vi "TDT-Wait For Buffer Space.vi"(0 "RPcox":refnum<k7>, 5 "Next Buffer":i32, 7 "Tag":string="ch2Index", 9 "Buffer Length":i32, 11 "error in (no error)":errorcluster, 12 "Timeout (ms)":i32=5000) -> (4 "RPcox Out":refnum<k7>, 6 "Next Buffer thru":i32, 15 "error out":errorcluster)   [LabVIEW 2020]
uses:
  TDT-Globals.vi
panel:
  out "Available":bool
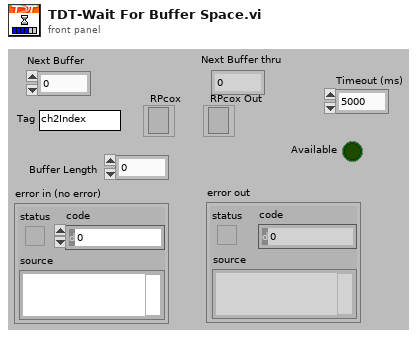
[diagram p1: front panel]
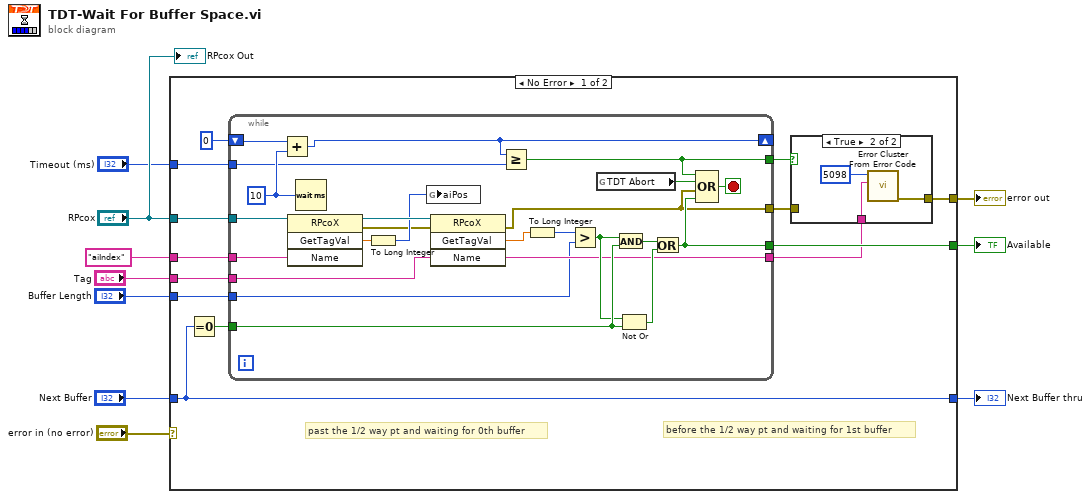
[diagram p0: block diagram]
diagram:
  n1 = case shown="No Error" "error in (no error)" {
    selector: "error in (no error)" -> [_ w52]
    tunnel: [w13 w52] -> w9
    tunnel: "RPcox" -> [w23 _]
    tunnel: "Buffer Length" -> [w22 _]
    tunnel: "Next Buffer" -> [w19 _]
    tunnel: [w20 _] -> w6
    tunnel: [w19 _] -> w5
    tunnel: "Tag" -> [w18 _]
    tunnel: "Timeout (ms)" -> [w16 _]
    tunnel: "aiIndex" ("format string") -> [w12 _]
    frame No Error {
      # "before the 1/2 way pt and waiting for 1st buffer"
      # "past the 1/2 way pt and waiting for 0th buffer"
      n2 = Equal To 0?(x=w19) -> (x = 0?=w21:bool)
      n3 = while {
        tunnel: w23 -> [w33]
        tunnel: w22 -> [w36]
        tunnel: w21 -> [w49]
        tunnel: [w45] -> w20
        tunnel: w18 -> [w43]
        shift-right: [w40] -> _
        shift-left: 0 -> [w42]
        tunnel: w16 -> [w39]
        tunnel: [w38] -> w15
        tunnel: [w37] -> w14
        tunnel: w12 -> [w32]
        tunnel: [w28] -> w11
        stop <- w44 stop-if-true
        w41 = u32 10 ("milliseconds to wait")
        n4 = Add(x=w42, y=w41) -> (x+y=w40:u32)
        n5 = invoke class="RPcoX" method="GetTagVal"(reference=w33, "Name"=w32) -> (reference out=w34:refnum<k7>, error out=w29:errorcluster, "GetTagVal"=w30:sgl)  [unwired: 2 in, 1 out]
        n6 = Wait (ms)(milliseconds to wait=w41) -> ()  [unwired: 1 out]
        n7 = To Long Integer(number=w30) -> (32bit integer=w31:i32)
        n8 = global write "TDT-Globals.vi" "aiPos"(w31) -> ()
        n9 = invoke class="RPcoX" method="GetTagVal"(reference=w34, error in=w29, "Name"=w43) -> (error out=w28:errorcluster, "GetTagVal"=w51:sgl, "Name"=w37:string)  [unwired: 1 in, 1 out]
        n10 = Greater Or Equal?(x=w40, y=w39) -> (x >= y?=w38:bool)
        n11 = To Long Integer(number=w51) -> (32bit integer=w35:i32)
        n12 = Greater?(x=w35, y=w36) -> (0:w48:bool)
        n13 = global read "TDT-Globals.vi" "TDT Abort"() -> (w46:bool)
        n14 = And(x=w48, y=w49) -> (x .and. y?=w50:bool)
        n15 = Not Or(1:w49, 2:w48) -> (0:w47:bool)
        n16 = Or(x=w50, y=w47) -> (x .or. y?=w45:bool)
        n17 = Compound Arithmetic op=OR(w38, w46, w28, w45) -> (w44:bool)
      }
      n18 = case shown="True" w15 {
        tunnel: w14 -> [_ w26]
        tunnel: [w24 w25] -> w13
        tunnel: w11 -> [w24 _]
        frame False {
        }
        frame True {
          n19 = call <vilib>:"Error Cluster From Error Code.vi"("error message (\"\")"=w26, "error code (0)"=5098 ("specific error code to clear (0: all)")) -> ("error out"=w25:errorcluster)  [unwired: 7 in]
        }
      }
    }
    frame Error {
    }
  }
  "error out" <- w9
  "Next Buffer thru" <- w5
  "Available" <- w6
  "RPcox Out" <- "RPcox"
